vi "main.vi"() -> ()   [LabVIEW 2016]
uses:
  <vilib>/Utility/config.llb/Read Key (I32).vi
  <vilib>/Utility/config.llb/Write Key (Double).vi
  <vilib>/Utility/config.llb/NI_LVConfig.lvlib
panel:
  out "说明":string
  in  "开始游戏":bool
  out "x/y":dbl
  in  "加速":dbl
  out "最高分":dbl
  out "分数":u32
  out "原等级":i8
  in  "等级":i8=4 min=1 max=10
  out "下一个":cluster{"编号":i8, "方块":i32[][]}
  out "当前":cluster{"编号":i8, "方块":i32[][]}
  out "下一个":picture
  out "数组":dbl[][](array[numeric])
  out "Game":bool
  in  "point":cluster{"x":i16, "y":i16} caption="当前位置"
  out "主界面":picture
  in  "主容器":dbl[][](array[numeric])
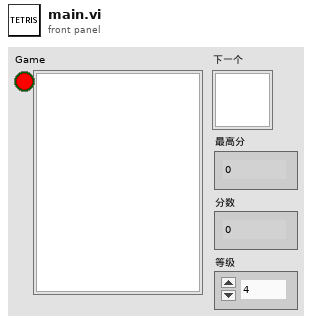
[diagram p1: front panel]
types:
  T1 = typedef "NI_LVConfig.lvlib/Config Data RefNum.ctl" = refnum<k1>
  T2 = typedef "imagedata.ctl" = cluster{"image type":i32, "image depth":i32, "image":u8[], "mask":u8[], "colors":u32[], "Rectangle":cluster{"left":i16, "top":i16, "right":i16, "bottom":i16}}
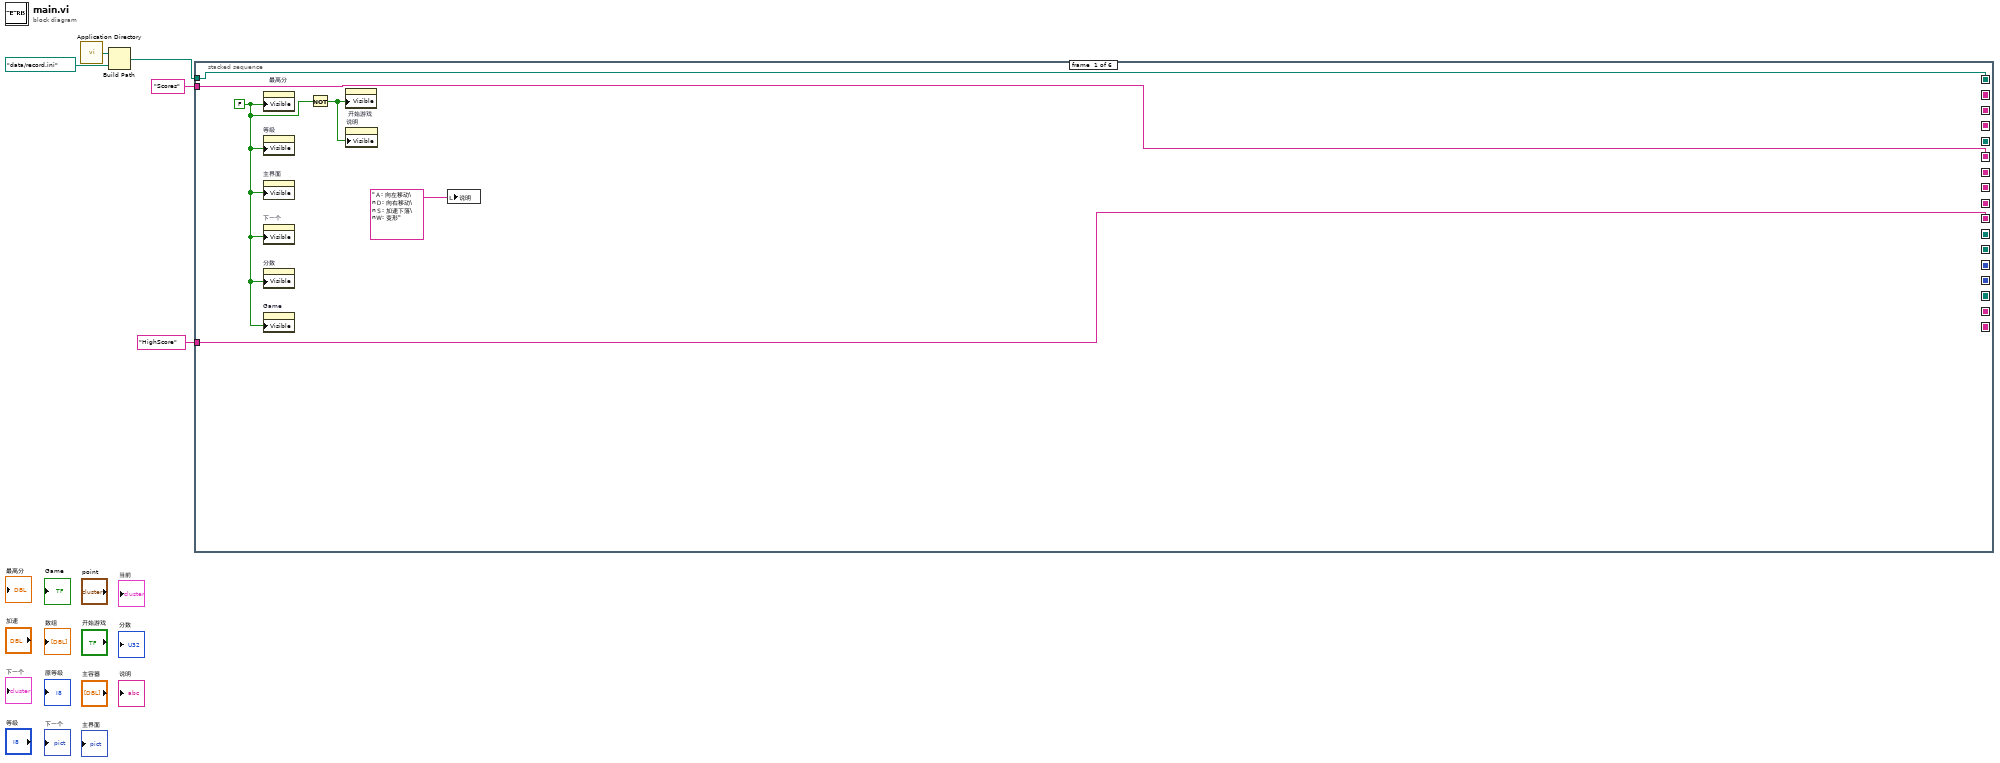
[diagram p0: block diagram]
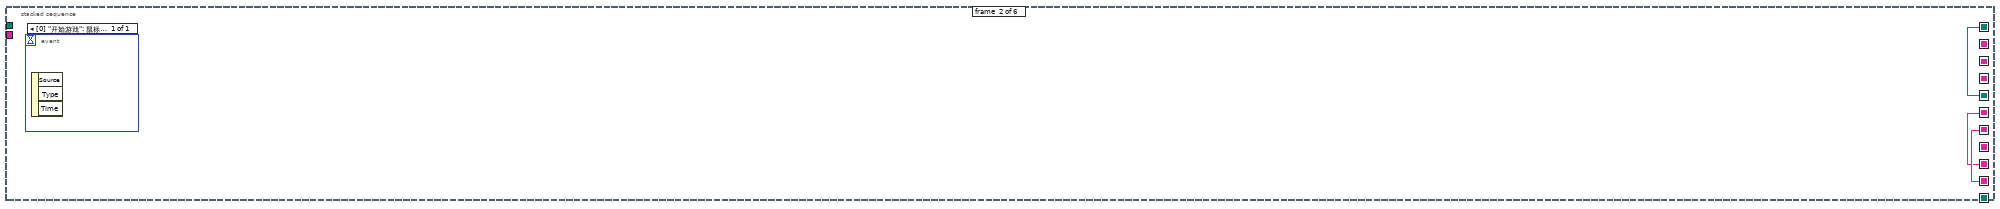
[diagram p2: hidden frame]
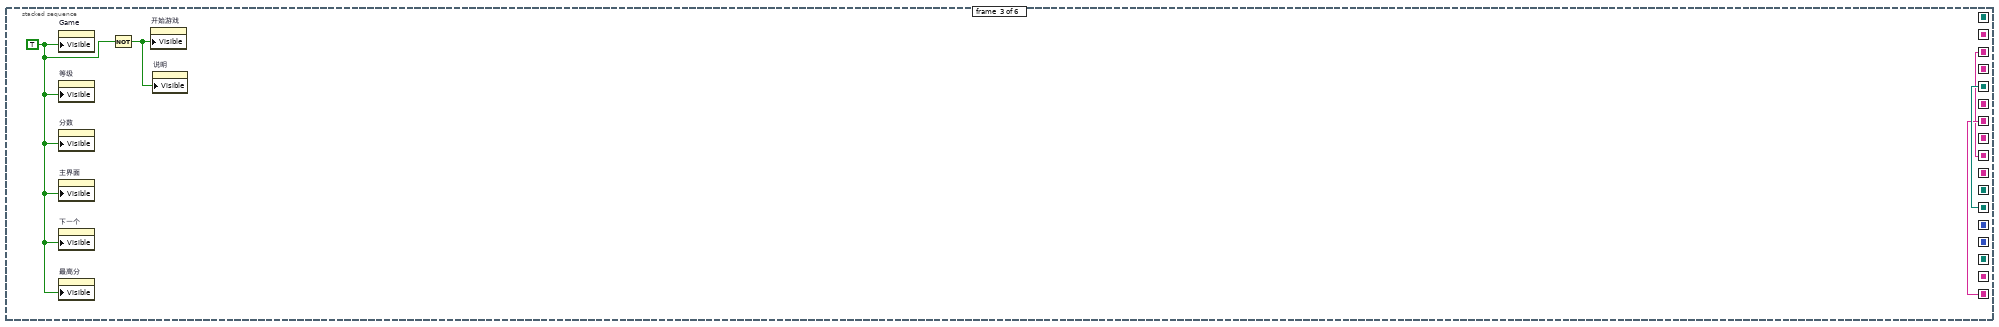
[diagram p3: hidden frame]
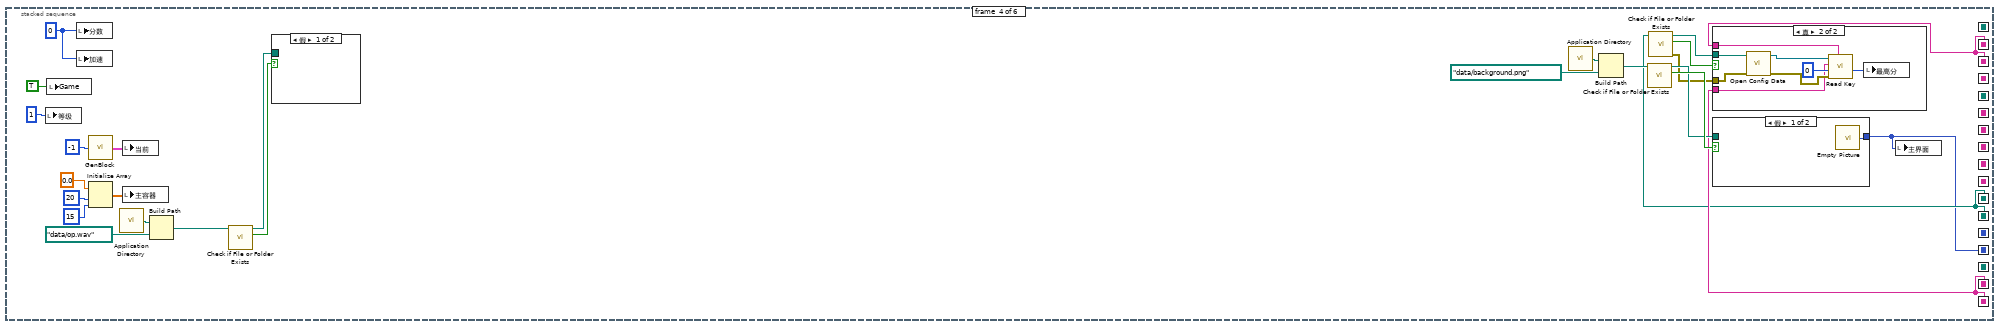
[diagram p4: hidden frame]
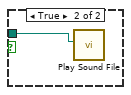
[diagram p6: hidden frame]
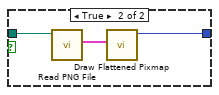
[diagram p7: hidden frame]
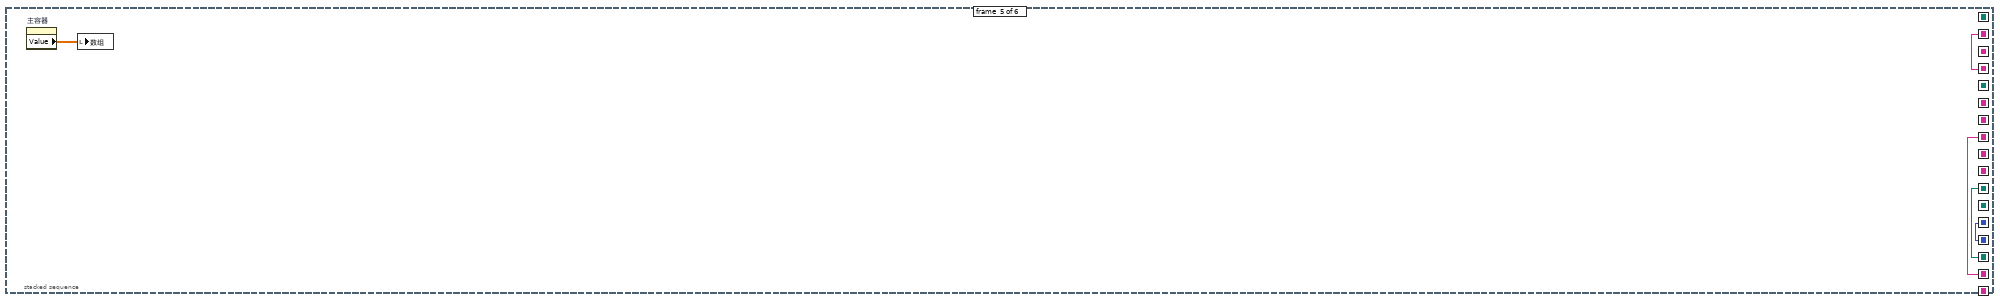
[diagram p8: hidden frame]
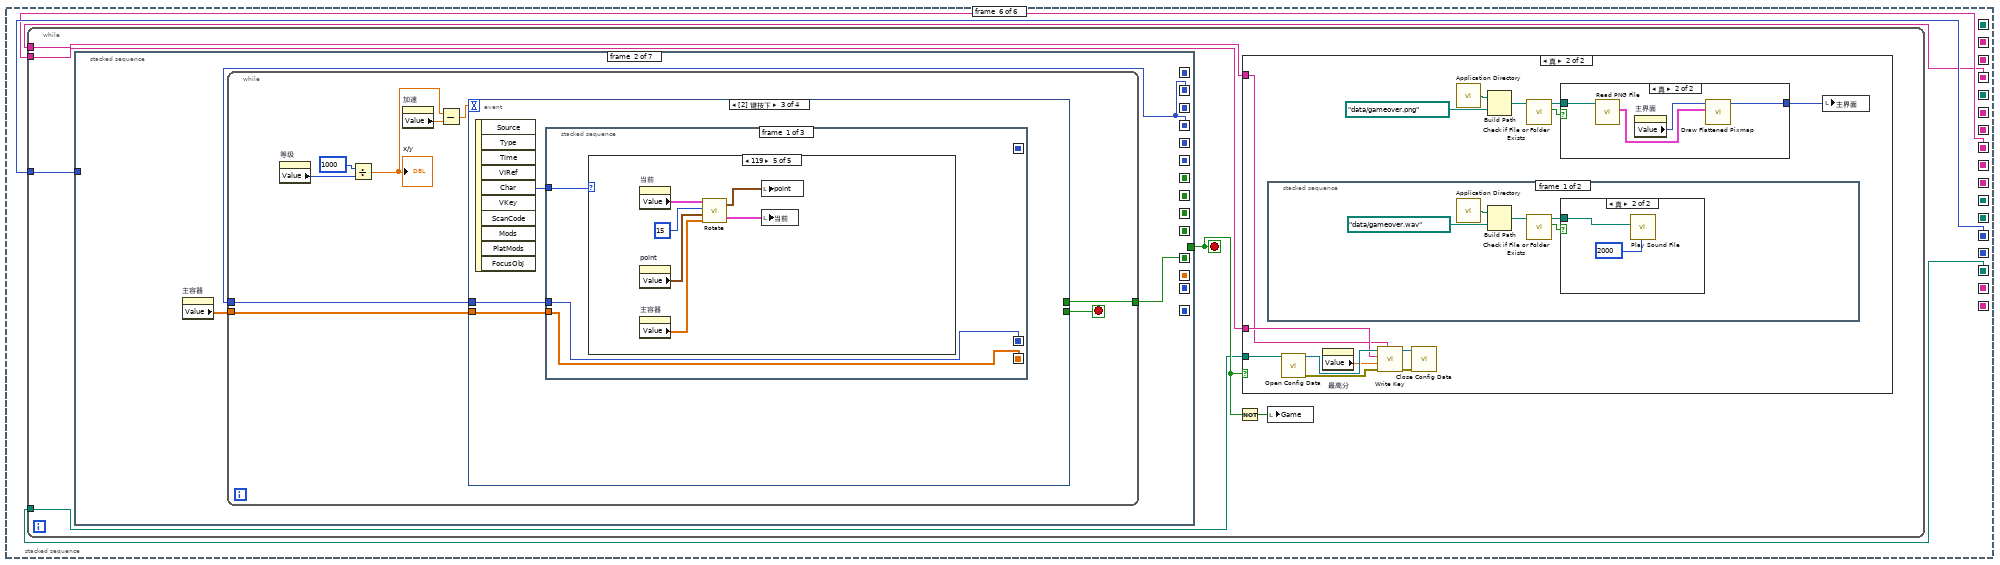
[diagram p9: hidden frame]
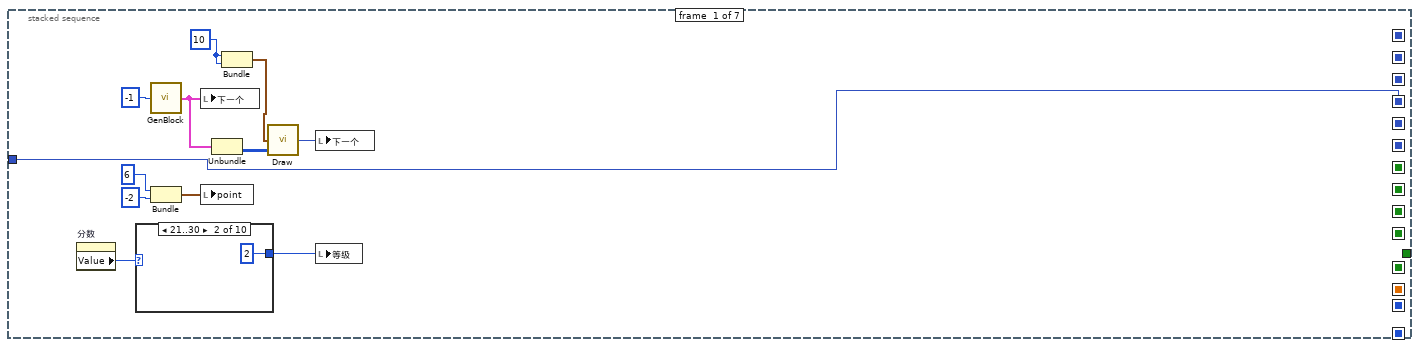
[diagram p10: hidden frame]
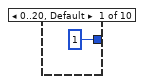
[diagram p11: hidden frame]
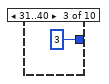
[diagram p12: hidden frame]
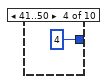
[diagram p13: hidden frame]
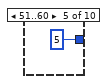
[diagram p14: hidden frame]
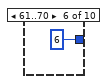
[diagram p15: hidden frame]
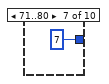
[diagram p16: hidden frame]
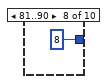
[diagram p17: hidden frame]
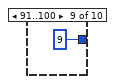
[diagram p18: hidden frame]
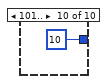
[diagram p19: hidden frame]
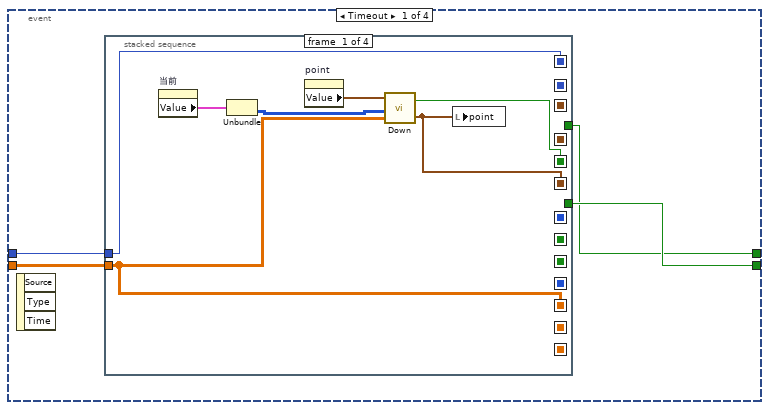
[diagram p20: hidden frame]
diagram:
  n1 = call <vilib>:"Application Directory.vi"() -> ("Application Directory"=w2:path)
  n2 = Build Path(base path=w2, name or relative path=path "data/record.ini") -> (appended path=w1:path)
  n3 = stacked-sequence {
    seq-local: [w11 _ _ _ _ _] -> [_ w14 _ _ _ _]
    seq-local: [w10 _ _ _ _ _] -> [_ w13 _ _ _ _]
    seq-local: [w9 _ _ _ _ _] -> [_ w12 _ _ _ _]
    seq-local: [_ w14 _ _ _ _] -> [_ _ w19 _ _ _]
    seq-local: [_ w13 _ _ _ _] -> [_ _ w18 _ _ _]
    seq-local: [_ w12 _ _ _ _] -> [_ _ w17 _ _ _]
    seq-local: [_ _ w19 _ _ _] -> [_ _ _ w22 _ _]
    seq-local: [_ _ w18 _ _ _] -> [_ _ _ w24 _ _]
    seq-local: [_ _ w17 _ _ _] -> [_ _ _ w23 _ _]
    seq-local: [_ _ _ w22 _ _] -> [_ _ _ _ w62 _]
    seq-local: [_ _ _ w24 _ _] -> [_ _ _ _ w61 _]
    seq-local: [_ _ _ w23 _ _] -> [_ _ _ _ w60 _]
    seq-local: [_ _ _ w20 _ _] -> [_ _ _ _ w59 _]
    seq-local: [_ _ _ _ w62 _] -> [_ _ _ _ _ w66]
    seq-local: [_ _ _ _ w61 _] -> [_ _ _ _ _ w65]
    seq-local: [_ _ _ _ w60 _] -> [_ _ _ _ _ w64]
    seq-local: [_ _ _ _ w59 _] -> [_ _ _ _ _ w67]
    tunnel: w1 -> [w11 _ _ _ _ _]
    tunnel: "HighScore" -> [w10 _ _ _ _ _]
    tunnel: "Scores" -> [w9 _ _ _ _ _]
    frame #0 {
      w8 = FALSE
      n4 = property on="最高分" class="DigNum (严格)"("Visible"=w8) -> ()  [unwired: 2 in, 2 out]
      n5 = property on="等级" class="DigNum (严格)"("Visible"=w8) -> ()  [unwired: 2 in, 2 out]
      n6 = property on="主界面" class="Pict"("Visible"=w8) -> ()  [unwired: 2 in, 2 out]
      n7 = property on="下一个" class="Pict"("Visible"=w8) -> ()  [unwired: 2 in, 2 out]
      n8 = property on="分数" class="DigNum (严格)"("Visible"=w8) -> ()  [unwired: 2 in, 2 out]
      n9 = property on="Game" class="Bool (严格)"("Visible"=w8) -> ()  [unwired: 2 in, 2 out]
      n10 = Not(x=w8) -> (.not. x?=w7:bool)
      n11 = property on="开始游戏" class="Bool (严格)"("Visible"=w7) -> ()  [unwired: 2 in, 2 out]
      n12 = property on="说明" class="Str"("Visible"=w7) -> ()  [unwired: 2 in, 2 out]
      n13 = local write "说明"("Ａ: 向左移动\nＤ: 向右移动\nＳ: 加速下落\nＷ: 变形") -> ()
    }
    frame #1 {
      n14 = event shown="[0] \"开始游戏\": 鼠标释放" {
        selector: _ -> [_]
        dyn-events: _ -> [_]
        timeout: _ -> [_]
        event "开始游戏": Mouse Up {
          n15 = event-data() -> ()  [unwired: 1 in, 3 out]
        }
      }
    }
    frame #2 {
      w16 = TRUE
      n16 = property on="Game" class="Bool (严格)"("Visible"=w16) -> ()  [unwired: 2 in, 2 out]
      n17 = property on="等级" class="DigNum (严格)"("Visible"=w16) -> ()  [unwired: 2 in, 2 out]
      n18 = property on="分数" class="DigNum (严格)"("Visible"=w16) -> ()  [unwired: 2 in, 2 out]
      n19 = property on="主界面" class="Pict"("Visible"=w16) -> ()  [unwired: 2 in, 2 out]
      n20 = property on="下一个" class="Pict"("Visible"=w16) -> ()  [unwired: 2 in, 2 out]
      n21 = property on="最高分" class="DigNum (严格)"("Visible"=w16) -> ()  [unwired: 2 in, 2 out]
      n22 = Not(x=w16) -> (.not. x?=w15:bool)
      n23 = property on="开始游戏" class="Bool (严格)"("Visible"=w15) -> ()  [unwired: 2 in, 2 out]
      n24 = property on="说明" class="Str"("Visible"=w15) -> ()  [unwired: 2 in, 2 out]
    }
    frame #3 {
      w21 = 0
      n25 = local write "等级"(1) -> ()
      n26 = local write "Game"(TRUE) -> ()
      n27 = local write "分数"(w21) -> ()
      n28 = local write "加速"(w21) -> ()
      n29 = call "GenBlock.vi"("编号"=-1) -> ("输出"=w39:cluster{"编号":i8, "方块":i32[][]})
      n30 = Initialize Array(0.0, 20, 15) -> (w45:dbl[][])
      n31 = call <vilib>:"Application Directory.vi"() -> ("Application Directory"=w29:path)
      n32 = local write "当前"(w39) -> ()
      n33 = local write "主容器"(w45) -> ()
      n34 = Build Path(base path=w29, name or relative path=path "data/op.wav") -> (appended path=w35:path)
      n35 = call <vilib>:"Check if File or Folder Exists.vi"("path"=w35) -> ("file or folder exists?"=w34:bool, "dup path"=w33:path)  [unwired: 8 in, 1 out]
      n36 = case shown="假" w34 {
        tunnel: w33 -> [_ w54]
        frame False {
        }
        frame True {
          n37 = call <vilib>:"Play Sound File.vi"("path"=w54) -> ()  [unwired: 9 in, 2 out]
        }
      }
      n38 = call <vilib>:"Application Directory.vi"() -> ("Application Directory"=w30:path)
      n39 = Build Path(base path=w30, name or relative path=path "data/background.png") -> (appended path=w36:path)
      n40 = call <vilib>:"Check if File or Folder Exists.vi"("path"=w36) -> ("file or folder exists?"=w38:bool, "dup path"=w37:path)  [unwired: 8 in, 1 out]
      n41 = call <vilib>:"Check if File or Folder Exists.vi"("path"=w22) -> ("error out"=w25:errorcluster, "file or folder exists?"=w27:bool, "dup path"=w26:path)  [unwired: 8 in]
      n42 = case shown="真" w27 {
        tunnel: w26 -> [_ w50]
        tunnel: w25 -> [_ w51]
        tunnel: w24 -> [_ w47]
        tunnel: w23 -> [_ w46]
        frame False {
        }
        frame True {
          n43 = call <vilib>:"Open Config Data.vi"("error in (no error)"=w51, "configuration file path"=w50) -> ("error out"=w53:errorcluster, "refnum"=w52:T1)  [unwired: 7 in, 1 out]
          n44 = call-poly <vilib>:"Read Key.vi"("section"=w46, "error in (no error)"=w53, "default value"=0, "key"=w47, "refnum"=w52) -> ("value"=w48:i32)  [unwired: 3 in, 3 out]
          n45 = local write "最高分"(w48) -> ()
        }
      }
      n46 = case shown="假" w38 {
        tunnel: [w55 w57] -> w20
        tunnel: w37 -> [_ w56]
        frame False {
          n47 = call "Empty Picture"() -> ("empty picture"=w55:picture)
        }
        frame True {
          n48 = call <vilib>:"Read PNG File.vi"("path to PNG file"=w56) -> ("image data"=w58:T2)  [unwired: 8 in, 2 out]
          n49 = call <vilib>:"Draw Flattened Pixmap.vi"("image data"=w58) -> ("new picture"=w57:picture)  [unwired: 8 in]
        }
      }
      n50 = local write "主界面"(w20) -> ()
    }
    frame #4 {
      n51 = property on="主容器" class="Arr (严格)"() -> ("Value"=w63:dbl[][])  [unwired: 2 in, 2 out]
      n52 = local write "数组"(w63) -> ()
    }
    frame #5 {
      n53 = while {
        tunnel: w67 -> [w73]
        tunnel: w66 -> [w71]
        tunnel: w65 -> [w70]
        tunnel: w64 -> [w69]
        stop <- w72 stop-if-true
        n54 = stacked-sequence {
          seq-local: [w79 _ _ _ _ _ _] -> [_ w96 _ _ _ _ _]
          seq-local: [_ w98 _ _ _ _ _] -> [_ _ w208 _ _ _ _]
          seq-local: [_ w96 _ _ _ _ _] -> [_ _ w207 _ _ _ _]
          seq-local: [_ _ w208 _ _ _ _] -> [_ _ _ w212 _ _ _]
          seq-local: [_ _ w207 _ _ _ _] -> [_ _ _ w211 _ _ _]
          seq-local: [_ _ _ w212 _ _ _] -> [_ _ _ _ w217 _ _]
          seq-local: [_ _ _ w214 _ _ _] -> [_ _ _ _ w221 _ _]
          seq-local: [_ _ _ w211 _ _ _] -> [_ _ _ _ w216 _ _]
          seq-local: [_ _ _ w213 _ _ _] -> [_ _ _ _ w218 _ _]
          seq-local: [_ _ _ _ w217 _ _] -> [_ _ _ _ _ w244 _]
          seq-local: [_ _ _ _ w221 _ _] -> [_ _ _ _ _ w245 _]
          seq-local: [_ _ _ _ w216 _ _] -> [_ _ _ _ _ w243 _]
          seq-local: [_ _ _ _ _ w244 _] -> [_ _ _ _ _ _ w251]
          seq-local: [_ _ _ _ _ w243 _] -> [_ _ _ _ _ _ w252]
          tunnel: w73 -> [w79 _ _ _ _ _ _]
          tunnel: [_ _ _ _ _ _ w251] -> w72
          frame #0 {
            w77 = 10
            n55 = property on="分数" class="DigNum (严格)"() -> ("Value"=w76:u32)  [unwired: 2 in, 2 out]
            n56 = case shown="21..30" w76 {
              tunnel: [1 2 3 4 5 6 7 8 9 10] -> w75
              frame 0..20, Default {
              }
              frame 21..30 {
              }
              frame 31..40 {
              }
              frame 41..50 {
              }
              frame 51..60 {
              }
              frame 61..70 {
              }
              frame 71..80 {
              }
              frame 81..90 {
              }
              frame 91..100 {
              }
              frame 101.. {
              }
            }
            n57 = call "GenBlock.vi"("编号"=-1) -> ("输出"=w80:cluster{"编号":i8, "方块":i32[][]})
            n58 = Bundle(6, -2) -> (w83:cluster{i32, i32})  [unwired: 1 in]
            n59 = local write "下一个"(w80) -> ()
            n60 = local write "point"(w83) -> ()
            n61 = Unbundle(w80) -> ("方块"=w81:i32[][])  [unwired: 1 out]
            n62 = Bundle(w77, w77) -> (w78:cluster{i32, i32})  [unwired: 1 in]
            n63 = call "Draw.vi"("数组"=w81, "point"=w78) -> ("输出"=w74:picture)  [unwired: 1 in]
            n64 = local write "下一个"(w74) -> ()
            n65 = local write "等级"(w75) -> ()
          }
          frame #1 {
            n66 = property on="主容器" class="Arr (严格)"() -> ("Value"=w97:dbl[][])  [unwired: 2 in, 2 out]
            n67 = while {
              tunnel: [w105] -> w98
              tunnel: w97 -> [w107]
              tunnel: w96 -> [w104]
              stop <- w106 stop-if-true
              n68 = property on="等级" class="DigNum (严格)"() -> ("Value"=w102:i8)  [unwired: 2 in, 2 out]
              n69 = Divide(x=1000, y=w102) -> (x/y=w101:dbl)
              "x/y" <- w101
              n70 = property on="加速" class="DigNum (严格)"() -> ("Value"=w100:dbl)  [unwired: 2 in, 2 out]
              n71 = Subtract(x=w101, y=w100) -> (x-y=w99:dbl)
              n72 = event shown="[2] 键按下" {
                selector: _ -> [_ _ _ _]
                dyn-events: _ -> [_ _ _ _]
                timeout: w99 -> [_ _ _ _]
                tunnel: w107 -> [w111 w141 w172 _]
                tunnel: [w110 _ _ _] -> w106
                tunnel: [w109 _ _ _] -> w105
                tunnel: w104 -> [w108 w140 w171 _]
                event Timeout {
                  n73 = event-data() -> ()  [unwired: 1 in, 3 out]
                  n74 = stacked-sequence {
                    seq-local: [w112 _ _ _] -> [_ w121 _ _]
                    seq-local: [w117 _ _ _] -> [_ w120 _ _]
                    seq-local: [w116 _ _ _] -> [_ w119 _ _]
                    seq-local: [w115 _ _ _] -> [_ w125 _ _]
                    seq-local: [_ w121 _ _] -> [_ _ w127 _]
                    seq-local: [_ w120 _ _] -> [_ _ w133 _]
                    seq-local: [_ w119 _ _] -> [_ _ w132 _]
                    seq-local: [_ w122 _ _] -> [_ _ w131 _]
                    seq-local: [_ w125 _ _] -> [_ _ w130 _]
                    seq-local: [_ _ w133 _] -> [_ _ _ w137]
                    seq-local: [_ _ w132 _] -> [_ _ _ w136]
                    seq-local: [_ _ w131 _] -> [_ _ _ w135]
                    seq-local: [_ _ w130 _] -> [_ _ _ w134]
                    tunnel: w111 -> [w115 _ _ _]
                    tunnel: w108 -> [w112 _ _ _]
                    tunnel: [_ _ _ w139] -> w109
                    tunnel: [_ _ _ w138] -> w110
                    frame #0 {
                      n75 = property on="当前" class="Clust (严格)"() -> ("Value"=w114:cluster{"编号":i8, "方块":i32[][]})  [unwired: 2 in, 2 out]
                      n76 = Unbundle(w114) -> ("方块"=w113:i32[][])  [unwired: 1 out]
                      n77 = property on="point" class="Clust (严格)"() -> ("Value"=w118:cluster{"x":i16, "y":i16})  [unwired: 2 in, 2 out]
                      n78 = call "Down.vi"("背景"=w115, "方块"=w113, "point"=w118) -> ("point 2"=w116:cluster{"x":i16, "y":i16}, "Landed"=w117:bool)
                      n79 = local write "point"(w116) -> ()
                    }
                    frame #1 {
                      n80 = property on="当前" class="Clust (严格)"() -> ("Value"=w123:cluster{"编号":i8, "方块":i32[][]})  [unwired: 2 in, 2 out]
                      n81 = Unbundle(w123) -> ("方块"=w122:i32[][])  [unwired: 1 out]
                      n82 = property on="point" class="Clust (严格)"() -> ("Value"=w126:cluster{"x":i16, "y":i16})  [unwired: 2 in, 2 out]
                      n83 = call "Merge.vi"("背景"=w125, "方块"=w122, "point"=w126) -> ("输出"=w124:u8[][])
                      n84 = local write "数组"(w124) -> ()
                    }
                    frame #2 {
                      n85 = property on="数组" class="Arr (严格)"() -> ("Value"=w128:dbl[][])  [unwired: 2 in, 2 out]
                      n86 = call "Draw.vi"("数组"=w128, "背景图片"=w127) -> ("输出"=w129:picture)  [unwired: 1 in]
                      n87 = local write "主界面"(w129) -> ()
                    }
                    frame #3 {
                      n88 = call "GameOver.vi"("背景"=w134, "方块"=w135, "point"=w136) -> ("输出"=w139:bool)
                      n89 = Or(x=w139, y=w137) -> (x .or. y?=w138:bool)
                    }
                  }
                }
                event Key Repeat {
                  n90 = event-data() -> ("Char"=w142:i16)  [unwired: 1 in, 9 out]
                  n91 = stacked-sequence {
                    seq-local: [w144 _ _] -> [_ w164 _]
                    seq-local: [w143 _ _] -> [_ w162 _]
                    seq-local: [_ w162 _] -> [_ _ w169]
                    tunnel: w142 -> [w145 _ _]
                    tunnel: w141 -> [w144 _ _]
                    tunnel: w140 -> [w143 _ _]
                    frame #0 {
                      n92 = case shown="100" w145 {
                        frame 0, Default {
                        }
                        frame 97 {
                          n93 = property on="当前" class="Clust (严格)"() -> ("Value"=w147:cluster{"编号":i8, "方块":i32[][]})  [unwired: 2 in, 2 out]
                          n94 = Unbundle(w147) -> ("方块"=w146:i32[][])  [unwired: 1 out]
                          n95 = property on="point" class="Clust (严格)"() -> ("Value"=w150:cluster{"x":i16, "y":i16})  [unwired: 2 in, 2 out]
                          n96 = property on="主容器" class="Arr (严格)"() -> ("Value"=w149:dbl[][])  [unwired: 2 in, 2 out]
                          n97 = call "Left.vi"("背景"=w149, "方块"=w146, "point"=w150) -> ("point 2"=w148:cluster{"x":i16, "y":i16})
                          n98 = local write "point"(w148) -> ()
                        }
                        frame 100 {
                          n99 = property on="当前" class="Clust (严格)"() -> ("Value"=w152:cluster{"编号":i8, "方块":i32[][]})  [unwired: 2 in, 2 out]
                          n100 = Unbundle(w152) -> ("方块"=w151:i32[][])  [unwired: 1 out]
                          n101 = property on="point" class="Clust (严格)"() -> ("Value"=w155:cluster{"x":i16, "y":i16})  [unwired: 2 in, 2 out]
                          n102 = property on="主容器" class="Arr (严格)"() -> ("Value"=w154:dbl[][])  [unwired: 2 in, 2 out]
                          n103 = call "Right.vi"("背景"=w154, "方块"=w151, "point"=w155) -> ("point 2"=w153:cluster{"x":i16, "y":i16})
                          n104 = local write "point"(w153) -> ()
                        }
                        frame 115 {
                        }
                        frame 119 {
                          n105 = property on="当前" class="Clust (严格)"() -> ("Value"=w160:cluster{"编号":i8, "方块":i32[][]})  [unwired: 2 in, 2 out]
                          n106 = property on="point" class="Clust (严格)"() -> ("Value"=w159:cluster{"x":i16, "y":i16})  [unwired: 2 in, 2 out]
                          n107 = property on="主容器" class="Arr (严格)"() -> ("Value"=w158:dbl[][])  [unwired: 2 in, 2 out]
                          n108 = call "Rotate.vi"("背景"=w158, "point"=w159, "宽度"=15, "输入"=w160) -> ("输出"=w161:cluster{"编号":i8, "方块":i32[][]}, "point 2"=w156:cluster{"x":i16, "y":i16})
                          n109 = local write "point"(w156) -> ()
                          n110 = local write "当前"(w161) -> ()
                        }
                      }
                    }
                    frame #1 {
                      n111 = property on="当前" class="Clust (严格)"() -> ("Value"=w166:cluster{"编号":i8, "方块":i32[][]})  [unwired: 2 in, 2 out]
                      n112 = Unbundle By Name(w166) -> ("方块"=w165:i32[][])
                      n113 = property on="point" class="Clust (严格)"() -> ("Value"=w167:cluster{"x":i16, "y":i16})  [unwired: 2 in, 2 out]
                      n114 = call "Merge.vi"("背景"=w164, "方块"=w165, "point"=w167) -> ("输出"=w163:u8[][])
                      n115 = local write "数组"(w163) -> ()
                    }
                    frame #2 {
                      n116 = property on="数组" class="Arr (严格)"() -> ("Value"=w170:dbl[][])  [unwired: 2 in, 2 out]
                      n117 = call "Draw.vi"("数组"=w170, "背景图片"=w169) -> ("输出"=w168:picture)  [unwired: 1 in]
                      n118 = local write "主界面"(w168) -> ()
                    }
                  }
                }
                event Key Down {
                  n119 = event-data() -> ("Char"=w173:i16)  [unwired: 1 in, 9 out]
                  n120 = stacked-sequence {
                    seq-local: [w175 _ _] -> [_ w198 _]
                    seq-local: [w174 _ _] -> [_ w196 _]
                    seq-local: [_ w196 _] -> [_ _ w203]
                    tunnel: w173 -> [w176 _ _]
                    tunnel: w172 -> [w175 _ _]
                    tunnel: w171 -> [w174 _ _]
                    frame #0 {
                      n121 = case shown="119" w176 {
                        frame 0, Default {
                        }
                        frame 97 {
                          n122 = property on="当前" class="Clust (严格)"() -> ("Value"=w178:cluster{"编号":i8, "方块":i32[][]})  [unwired: 2 in, 2 out]
                          n123 = Unbundle(w178) -> ("方块"=w177:i32[][])  [unwired: 1 out]
                          n124 = property on="point" class="Clust (严格)"() -> ("Value"=w181:cluster{"x":i16, "y":i16})  [unwired: 2 in, 2 out]
                          n125 = property on="主容器" class="Arr (严格)"() -> ("Value"=w180:dbl[][])  [unwired: 2 in, 2 out]
                          n126 = call "Left.vi"("背景"=w180, "方块"=w177, "point"=w181) -> ("point 2"=w179:cluster{"x":i16, "y":i16})
                          n127 = local write "point"(w179) -> ()
                        }
                        frame 100 {
                          n128 = property on="当前" class="Clust (严格)"() -> ("Value"=w183:cluster{"编号":i8, "方块":i32[][]})  [unwired: 2 in, 2 out]
                          n129 = Unbundle(w183) -> ("方块"=w182:i32[][])  [unwired: 1 out]
                          n130 = property on="point" class="Clust (严格)"() -> ("Value"=w186:cluster{"x":i16, "y":i16})  [unwired: 2 in, 2 out]
                          n131 = property on="主容器" class="Arr (严格)"() -> ("Value"=w185:dbl[][])  [unwired: 2 in, 2 out]
                          n132 = call "Right.vi"("背景"=w185, "方块"=w182, "point"=w186) -> ("point 2"=w184:cluster{"x":i16, "y":i16})
                          n133 = local write "point"(w184) -> ()
                        }
                        frame 115 {
                          n134 = property on="x/y" class="DigNum (严格)"() -> ("Value"=w189:dbl)  [unwired: 2 in, 2 out]
                          n135 = Subtract(x=w189, y=10) -> (x-y=w187:dbl)
                          n136 = local write "加速"(w187) -> ()
                        }
                        frame 119 {
                          n137 = property on="当前" class="Clust (严格)"() -> ("Value"=w194:cluster{"编号":i8, "方块":i32[][]})  [unwired: 2 in, 2 out]
                          n138 = property on="point" class="Clust (严格)"() -> ("Value"=w193:cluster{"x":i16, "y":i16})  [unwired: 2 in, 2 out]
                          n139 = property on="主容器" class="Arr (严格)"() -> ("Value"=w192:dbl[][])  [unwired: 2 in, 2 out]
                          n140 = call "Rotate.vi"("背景"=w192, "point"=w193, "宽度"=15, "输入"=w194) -> ("输出"=w195:cluster{"编号":i8, "方块":i32[][]}, "point 2"=w190:cluster{"x":i16, "y":i16})
                          n141 = local write "point"(w190) -> ()
                          n142 = local write "当前"(w195) -> ()
                        }
                      }
                    }
                    frame #1 {
                      n143 = property on="当前" class="Clust (严格)"() -> ("Value"=w200:cluster{"编号":i8, "方块":i32[][]})  [unwired: 2 in, 2 out]
                      n144 = Unbundle By Name(w200) -> ("方块"=w199:i32[][])
                      n145 = property on="point" class="Clust (严格)"() -> ("Value"=w201:cluster{"x":i16, "y":i16})  [unwired: 2 in, 2 out]
                      n146 = call "Merge.vi"("背景"=w198, "方块"=w199, "point"=w201) -> ("输出"=w197:u8[][])
                      n147 = local write "数组"(w197) -> ()
                    }
                    frame #2 {
                      n148 = property on="数组" class="Arr (严格)"() -> ("Value"=w204:dbl[][])  [unwired: 2 in, 2 out]
                      n149 = call "Draw.vi"("数组"=w204, "背景图片"=w203) -> ("输出"=w202:picture)  [unwired: 1 in]
                      n150 = local write "主界面"(w202) -> ()
                    }
                  }
                }
                event Key Up {
                  n151 = event-data() -> ("ScanCode"=w205:i16)  [unwired: 1 in, 7 out]
                  n152 = case shown="31" w205 {
                    frame 0, Default {
                    }
                    frame 31 {
                      n153 = local write "加速"(0) -> ()
                    }
                  }
                }
              }
            }
          }
          frame #2 {
            n154 = property on="下一个" class="Clust (严格)"() -> ("Value"=w209:cluster{"编号":i8, "方块":i32[][]})  [unwired: 2 in, 2 out]
            n155 = property on="数组" class="Arr (严格)"() -> ("Value"=w210:dbl[][])  [unwired: 2 in, 2 out]
            n156 = local write "当前"(w209) -> ()
            n157 = local write "主容器"(w210) -> ()
          }
          frame #3 {
            n158 = property on="主容器" class="Arr (严格)"() -> ("Value"=w215:dbl[][])  [unwired: 2 in, 2 out]
            n159 = call "Clear.vi"("输入"=w215) -> ("清除行"=w214:i16[], "得分"=w213:dbl)  [unwired: 1 in]
          }
          frame #4 {
            n160 = property on="分数" class="DigNum (严格)"() -> ("Value"=w220:u32)  [unwired: 2 in, 2 out]
            n161 = case shown="4" w218 {
              frame 0, Default {
              }
              frame 1..3 {
                n162 = call <vilib>:"Application Directory.vi"() -> ("Application Directory"=w223:path)
                n163 = Build Path(base path=w223, name or relative path=path "data/clear.wav") -> (appended path=w224:path)
                n164 = call <vilib>:"Check if File or Folder Exists.vi"("path"=w224) -> ("file or folder exists?"=w225:bool, "dup path"=w226:path)  [unwired: 8 in, 1 out]
                n165 = case shown="真" w225 {
                  tunnel: w226 -> [_ w227]
                  frame False {
                  }
                  frame True {
                    n166 = call <vilib>:"Play Sound File.vi"("path"=w227) -> ()  [unwired: 9 in, 2 out]
                  }
                }
              }
              frame 4 {
                n167 = property on="分数" class="DigNum (严格)"() -> ("Value"=w230:u32)  [unwired: 2 in, 2 out]
                n168 = Add(x=10, y=w230) -> (x+y=w229:u32)
                n169 = local write "分数"(w229) -> ()
                n170 = call <vilib>:"Application Directory.vi"() -> ("Application Directory"=w232:path)
                n171 = Build Path(base path=w232, name or relative path=path "data/boom.wav") -> (appended path=w233:path)
                n172 = call <vilib>:"Check if File or Folder Exists.vi"("path"=w233) -> ("file or folder exists?"=w234:bool, "dup path"=w235:path)  [unwired: 8 in, 1 out]
                n173 = case shown="真" w234 {
                  tunnel: w235 -> [_ w236]
                  frame False {
                  }
                  frame True {
                    n174 = call <vilib>:"Play Sound File.vi"("path"=w236) -> ()  [unwired: 9 in, 2 out]
                  }
                }
              }
            }
            n175 = Add(x=w220, y=w218) -> (x+y=w219:dbl)
            n176 = local write "分数"(w219) -> ()
            n177 = for {
              tunnel: w221 -> [w239] mode=indexing
              n178 = property on="主容器" class="Arr (严格)"() -> ("Value"=w238:dbl[][])  [unwired: 2 in, 2 out]
              n179 = Delete From Array(array=w238, index (row)=w239) -> (array with subset deleted=w237:dbl[][])  [unwired: 2 in, 1 out]
              n180 = local write "主容器"(w237) -> ()
            }
          }
          frame #5 {
            n181 = property on="最高分" class="DigNum (严格)"() -> ("Value"=w240:dbl)  [unwired: 2 in, 2 out]
            n182 = property on="分数" class="DigNum (严格)"() -> ("Value"=w242:u32)  [unwired: 2 in, 2 out]
            n183 = Max & Min(x=w240, y=w242) -> (max(x,y)=w241:dbl)  [unwired: 1 out]
            n184 = local write "最高分"(w241) -> ()
            n185 = for {
              tunnel: w245 -> [_] mode=indexing
              w249 = 0
              n186 = Initialize Array(w249, 15) -> (w250:i32[])
              n187 = property on="主容器" class="Arr (严格)"() -> ("Value"=w247:dbl[][])  [unwired: 2 in, 2 out]
              n188 = Insert Into Array(array=w247, index (row)=w249, new element=w250) -> (w246:dbl[][])  [unwired: 1 in]
              n189 = local write "主容器"(w246) -> ()
            }
          }
          frame #6 {
            n190 = property on="主容器" class="Arr (严格)"() -> ("Value"=w254:dbl[][])  [unwired: 2 in, 2 out]
            n191 = call "Draw.vi"("数组"=w254, "背景图片"=w252) -> ("输出"=w253:picture)  [unwired: 1 in]
            n192 = local write "主界面"(w253) -> ()
          }
        }
        n193 = Not(x=w72) -> (.not. x?=w68:bool)
        n194 = case shown="真" w72 {
          tunnel: w71 -> [_ w262]
          tunnel: w70 -> [_ w260]
          tunnel: w69 -> [_ w259]
          frame False {
          }
          frame True {
            n195 = stacked-sequence {
              frame #0 {
                n196 = call <vilib>:"Application Directory.vi"() -> ("Application Directory"=w272:path)
                n197 = Build Path(base path=w272, name or relative path=path "data/gameover.wav") -> (appended path=w271:path)
                n198 = call <vilib>:"Check if File or Folder Exists.vi"("path"=w271) -> ("file or folder exists?"=w270:bool, "dup path"=w269:path)  [unwired: 8 in, 1 out]
                n199 = case shown="真" w270 {
                  tunnel: w269 -> [_ w275]
                  frame False {
                  }
                  frame True {
                    n200 = call <vilib>:"Play Sound File.vi"("timeout (sec)"=2000, "path"=w275) -> ()  [unwired: 8 in, 2 out]
                  }
                }
              }
              frame #1 {
                n201 = call <vilib>:"Application Directory.vi"() -> ("Application Directory"=w278:path)
                n202 = Build Path(base path=w278, name or relative path=path "data/background.png") -> (appended path=w280:path)
                n203 = call <vilib>:"Check if File or Folder Exists.vi"("path"=w280) -> ("file or folder exists?"=w277:bool, "dup path"=w276:path)  [unwired: 8 in, 1 out]
                n204 = case shown="真" w277 {
                  tunnel: w276 -> [_ w283]
                  frame False {
                  }
                  frame True {
                    n205 = call <vilib>:"Read PNG File.vi"("path to PNG file"=w283) -> ("image data"=w282:T2)  [unwired: 8 in, 2 out]
                    n206 = call <vilib>:"Draw Flattened Pixmap.vi"("image data"=w282) -> ("new picture"=w281:picture)  [unwired: 8 in]
                    n207 = local write "主界面"(w281) -> ()
                  }
                }
              }
            }
            n208 = call <vilib>:"Open Config Data.vi"("configuration file path"=w262) -> ("error out"=w257:errorcluster, "refnum"=w261:T1)  [unwired: 8 in, 1 out]
            n209 = property on="最高分" class="DigNum (严格)"() -> ("Value"=w258:dbl)  [unwired: 2 in, 2 out]
            n210 = call-poly <vilib>:"Write Key.vi"("section"=w259, "error in (no error)"=w257, "value"=w258, "key"=w260, "refnum"=w261) -> ("error out"=w255:errorcluster, "refnum out"=w256:T1)  [unwired: 4 in, 1 out]
            n211 = call <vilib>:"Close Config Data.vi"("error in (no error)"=w255, "refnum"=w256) -> ()  [unwired: 8 in, 2 out]
            n212 = call <vilib>:"Application Directory.vi"() -> ("Application Directory"=w268:path)
            n213 = Build Path(base path=w268, name or relative path=path "data/gameover.png") -> (appended path=w266:path)
            n214 = call <vilib>:"Check if File or Folder Exists.vi"("path"=w266) -> ("file or folder exists?"=w264:bool, "dup path"=w265:path)  [unwired: 8 in, 1 out]
            n215 = case shown="真" w264 {
              tunnel: w265 -> [_ w287]
              tunnel: [w284 w285] -> w263
              frame False {
                n216 = call "Empty Picture"() -> ("empty picture"=w284:picture)
              }
              frame True {
                n217 = call <vilib>:"Read PNG File.vi"("path to PNG file"=w287) -> ("image data"=w288:T2)  [unwired: 8 in, 2 out]
                n218 = property on="主界面" class="Pict"() -> ("Value"=w286:picture)  [unwired: 2 in, 2 out]
                n219 = call <vilib>:"Draw Flattened Pixmap.vi"("image data"=w288, "picture"=w286) -> ("new picture"=w285:picture)  [unwired: 7 in]
              }
            }
            n220 = local write "主界面"(w263) -> ()
          }
        }
        n221 = local write "Game"(w68) -> ()
      }
    }
  }
